vi "Configure Output.vi"(8 "error in (no error)":errorcluster, 9 "Voltage Level (0.00 V)":dbl format="%.2g", 10 "Enable Output (T: Enable)":bool=TRUE, 11 "VISA resource name":refnum<visa-resource-name>) -> (0 "error out":errorcluster, 1 "Voltage level":string, 3 "VISA resource name out":refnum<visa-resource-name>)   [LabVIEW 2020]
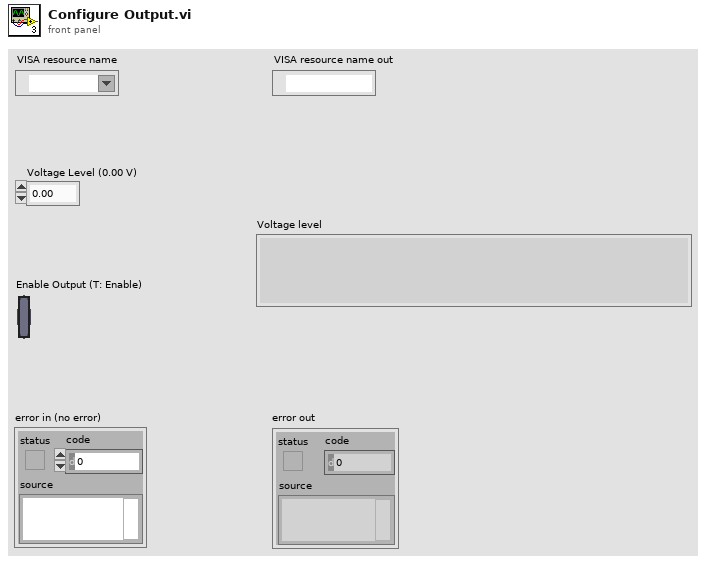
[diagram p1: front panel]
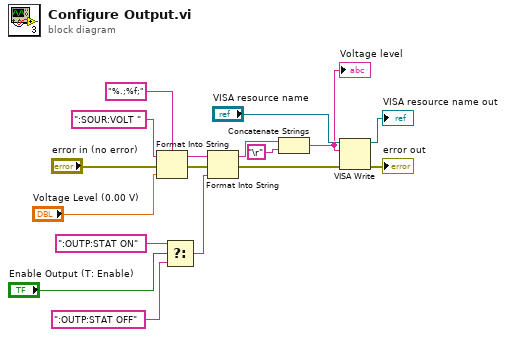
[diagram p0: block diagram]
diagram:
  n1 = Format Into String(format string="%.;%f;", initial string=":SOUR:VOLT ", error in="error in (no error)", "Voltage Level (0.00 V)") -> (resulting string=w10:string, error out=w1:errorcluster)
  n2 = Select(t=":OUTP:STAT ON", s="Enable Output (T: Enable)", f=":OUTP:STAT OFF") -> (s? t:f=w9:string)
  n3 = Format Into String(initial string=w10, error in=w1, w9) -> (resulting string=w6:string, error out=w2:errorcluster)  [unwired: 1 in]
  n4 = Concatenate Strings(w6, "\r") -> (w5:string)
  "Voltage level" <- w5
  n5 = VISA Write(VISA resource name="VISA resource name", write buffer=w5, error in (no error)=w2) -> (VISA resource name out=→"VISA resource name out":refnum<visa-resource-name>, error out=→"error out":errorcluster)  [unwired: 1 out]
